vi "Toggle Visibility.vi"(8 "error in (no error)":errorcluster, 10 "This VI":refnum<vi>, 11 "SubPanel in":refnum<vi>) -> (0 "error out":errorcluster)   [LabVIEW 2019, in "Peek Window.lvlib"]
uses:
  Peek Window.lvlib
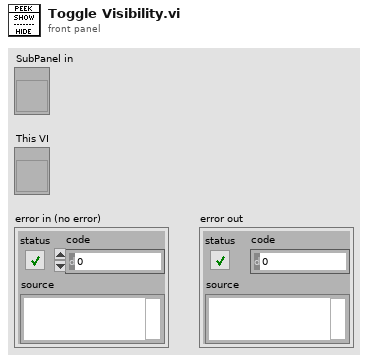
[diagram p1: front panel]
types:
  T1 = enum32{"Invalid", "Standard", "Closed", "Hidden", "Minimized", "Maximized"}
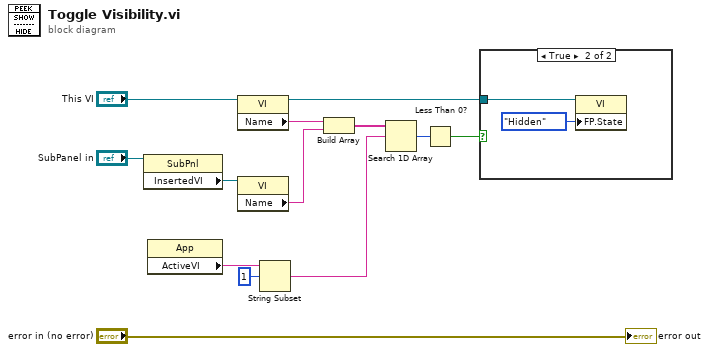
[diagram p0: block diagram]
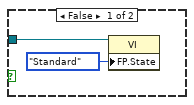
[diagram p2: hidden frame]
diagram:
  n1 = property class="SubPnl"(reference="SubPanel in") -> ("InsertedVI"=w11:refnum<vi>)  [unwired: 1 in, 2 out]
  n2 = property class="App"() -> ("ActiveVI"=w9:string)  [unwired: 2 in, 2 out]
  n3 = property class="VI"(reference="This VI") -> (reference out=w1:refnum<vi>, "Name"=w7:string)  [unwired: 1 in, 1 out]
  n4 = property class="VI"(reference=w11) -> ("Name"=w6:string)  [unwired: 1 in, 2 out]
  n5 = String Subset(string=w9, offset (0)=1) -> (substring=w4:string)  [unwired: 1 in]
  n6 = Build Array(w7, w6) -> (w5:string[])
  n7 = Search 1D Array(1D array=w5, element=w4) -> (index of element=w3:i32)  [unwired: 1 in]
  n8 = Less Than 0?(x=w3) -> (x < 0?=w2:bool)
  n9 = case shown="True" w2 {
    tunnel: w1 -> [w14 w17]
    frame False {
      n10 = property class="VI"(reference=w14, "FP.State"=T1."Standard" ("Front Panel Window:State")) -> ()  [unwired: 1 in, 2 out]
    }
    frame True {
      n11 = property class="VI"(reference=w17, "FP.State"=T1."Hidden" ("Front Panel Window:State")) -> ()  [unwired: 1 in, 2 out]
    }
  }
  "error out" <- "error in (no error)"
